vi "Apply System Image.vi"(7 "Installation Notifiers":T1, 8 "error in":errorcluster caption="error in (no error)", 11 "Target settings":T2={"Hostname"="", "Serial number"="", "Product name"="", "Product code"=0, "System status"="", "Credential type"=enum."None/Unlocked", "User added?"=FALSE, "Primary NIC"={"MAC address"="", "IP Address Request Mode"=2, "IP address"="", "Subnet mask"="", "Gateway"="", "DNS server"=""}, "System Credentials"={"Username"="", "Password"=""}} {"Primary NIC"."IP Address Request Mode" items=["Static"=1, "DHCP/Link-Local"=2, "Link-Local Only"=4, "DHCP Only"=8]}) -> (0 "error out":errorcluster, 3 "Real-Time:System Status":string)   [LabVIEW 2020]
doc: "Applies the most updated system image found in the local machine."
uses:
  Controls/Target Information.ctl
  Controls/Target Network Settings.ctl
  Controls/System Credentials.ctl
  Controls/Installation Notifiers.ctl
  Controls/Deployment Status Data Type.ctl
  Controls/Deployment Progress Data Type.ctl
  <vilib>/nisyscfg/Network Settings Format.ctl
  <vilib>/nisyscfg/Format With Base System Image.vi
  <vilib>/nisyscfg/Close (System).vi
  <vilib>/nisyscfg/nisyscfg.lvlib
  <resource>/objmgr/nisysapi.rc
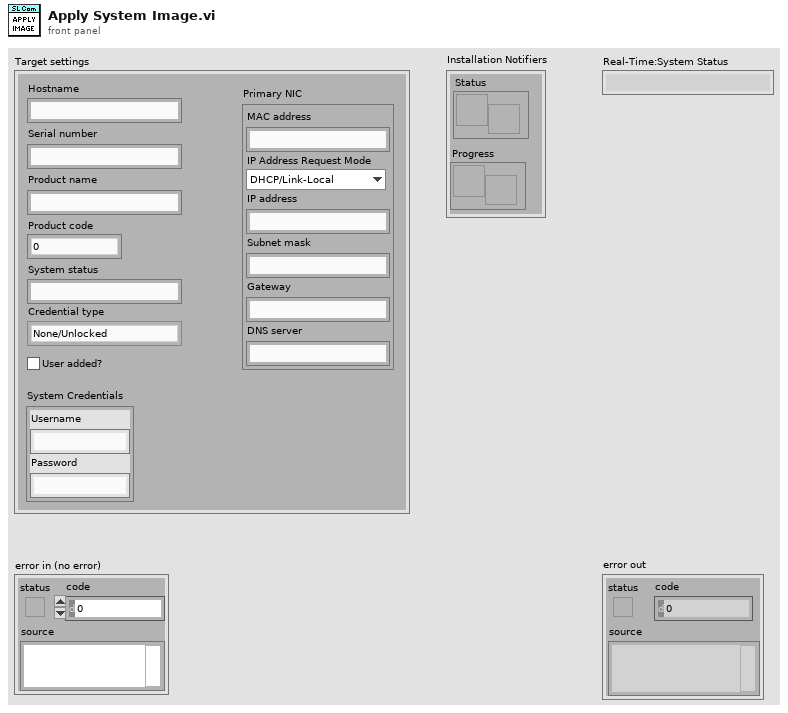
[diagram p1: front panel]
types:
  T1 = typedef "Installation Notifiers.ctl" = cluster{"Status":refnum<notifier>, "Progress":refnum<notifier>}
  T2 = typedef "Target Information.ctl" = cluster{"Hostname":string, "Serial number":string, "Product name":string, "Product code":i32, "System status":string, "Credential type":enum16{"None/Unlocked", "FTP Password", "NIAuth Credentials"}, "User added?":bool, "Primary NIC":T3, "System Credentials":T4}
  T3 = typedef "Target Network Settings.ctl" = cluster{"MAC address":string, "IP Address Request Mode":i32, "IP address":string, "Subnet mask":string, "Gateway":string, "DNS server":string}
  T4 = typedef "System Credentials.ctl" = cluster{"Username":string, "Password":string}
  T5 = typedef "Deployment Progress Data Type.ctl" = i8
  T6 = typedef "Deployment Status Data Type.ctl" = string
  T7 = typedef "nisyscfg.lvlib/Network Settings Format.ctl" = u32
  T8 = typedef "nisyscfg.lvlib/Software 1.2.ctl" = cluster{"title":string, "description":string, "ID":string, "version":string, "component type":T9}
  T9 = typedef "nisyscfg.lvlib/Component Type.ctl" = u32
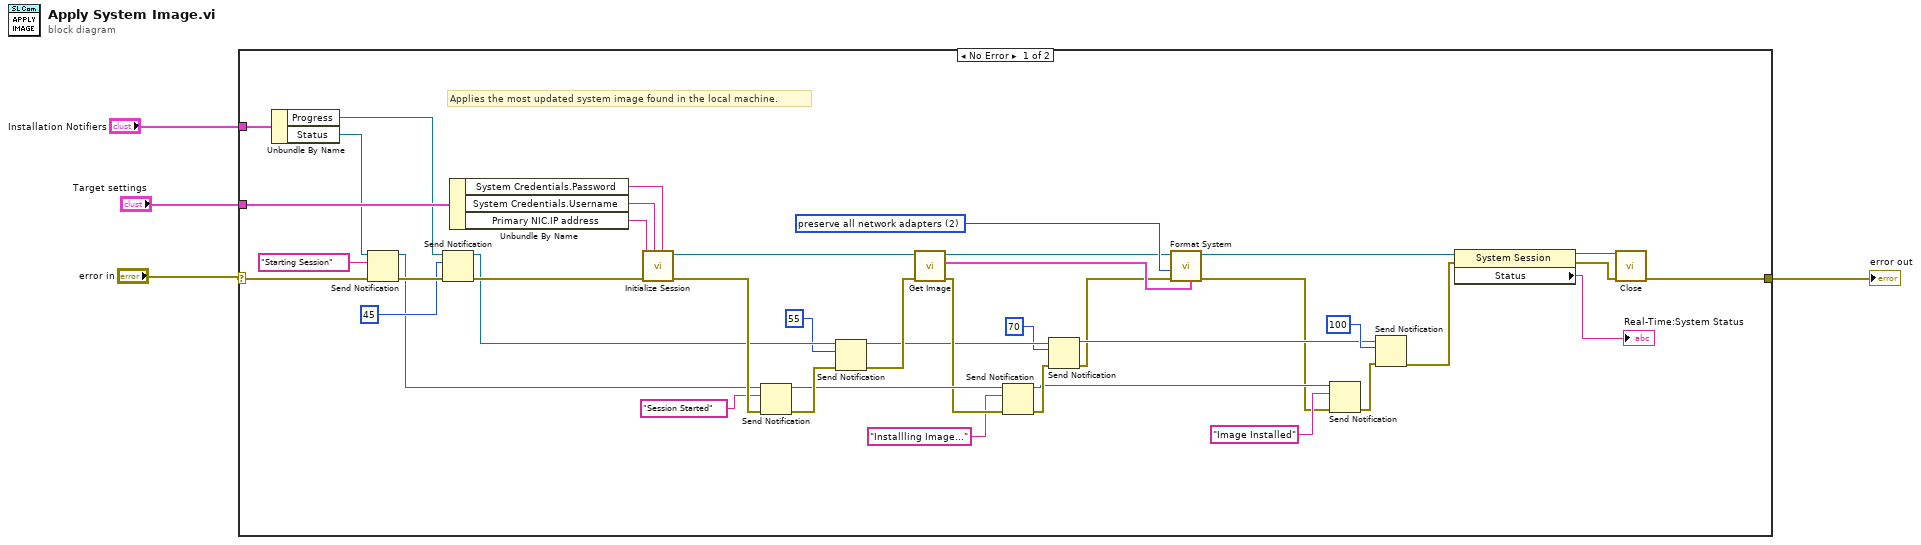
[diagram p0: block diagram]
diagram:
  n1 = case shown="No Error" "error in" {
    selector: "error in" -> [w43 w47]
    tunnel: [w46 w47] -> w2
    tunnel: "Target settings" -> [w45 _]
    tunnel: "Installation Notifiers" -> [w32 _]
    frame No Error {
      w42 = T7 2 items=["reset all network adapters", "preserve primary, reset others", "preserve all network adapters"] ("Network Settings (reset all adapters)")
      # "Applies the most updated system image found in the local machine."
      n2 = Unbundle By Name(w32) -> ("Progress"=w28:refnum<notifier>, "Status"=w29:refnum<notifier>)
      n3 = Send Notification(notification=T6 "Starting Session", notifier=w29, error in (no error)=w43) -> (notifier out=w23:refnum<notifier>, error out=w30:errorcluster)
      n4 = Send Notification(notification=T5 45, notifier=w28, error in (no error)=w30) -> (notifier out=w21:refnum<notifier>, error out=w31:errorcluster)
      n5 = Unbundle By Name(w45) -> ("System Credentials.Password"=w33:string, "System Credentials.Username"=w34:string, "Primary NIC.IP address"=w44:string)
      n6 = call <vilib>:"Initialize Session.vi"("Password"=w33, "User Name"=w34, "error in (no error)"=w31, "Target (localhost)"=w44) -> ("error out"=w24:errorcluster, "Session out"=w41:refnum<k21>)  [unwired: 6 in]
      n7 = Send Notification(notification=T6 "Session Started", notifier=w23, error in (no error)=w24) -> (notifier out=w18:refnum<notifier>, error out=w25:errorcluster)
      n8 = Send Notification(notification=T5 55, notifier=w21, error in (no error)=w25) -> (notifier out=w16:refnum<notifier>, error out=w19:errorcluster)
      n9 = call "Get Image.vi"("error in"=w19, "Refnum in"=w41) -> ("error out"=w17:errorcluster, "element"=w39:T8, "Refnum out"=w40:refnum<k21>)  [unwired: 7 in]
      n10 = Send Notification(notification=T6 "Installling Image...", notifier=w18, error in (no error)=w17) -> (notifier out=w8:refnum<notifier>, error out=w15:errorcluster)
      n11 = Send Notification(notification=T5 70, notifier=w16, error in (no error)=w15) -> (notifier out=w9:refnum<notifier>, error out=w7:errorcluster)
      n12 = call-poly <vilib>:"Format System.vi"("Base System Image"=w39, "error in (no error)"=w7, "Network Settings (reset all adapters)"=w42, "Session in"=w40) -> ("error out"=w6:errorcluster, "Session out"=w38:refnum<k21>)  [unwired: 6 in]
      n13 = Send Notification(notification=T6 "Image Installed", notifier=w8, error in (no error)=w6) -> (error out=w10:errorcluster)  [unwired: 1 out]
      n14 = Send Notification(notification=T5 100, notifier=w9, error in (no error)=w10) -> (error out=w5:errorcluster)  [unwired: 1 out]
      n15 = property class="System Session"(reference=w38, error in=w5) -> (reference out=w37:refnum<k21>, error out=w36:errorcluster, "Status"=→"Real-Time:System Status":string)
      n16 = call-poly <vilib>:"Close.vi"("error in (no error)"=w36, "Session in"=w37) -> ("error out"=w46:errorcluster)  [unwired: 9 in]
    }
    frame Error {
    }
  }
  "error out" <- w2
